vi "Print VI panel to PDF.vi"(6 "jobIndex (0)":i32, 7 "Entire Panel? (T)":bool=TRUE, 8 "error in":errorcluster, 9 "Time out (3 sec)":i32=3, 10 "VI in":refnum<vi>, 11 "path":path) -> (0 "error out":errorcluster, 2 "IsSuccessful":bool, 3 "path out":path)   [LabVIEW 2020]
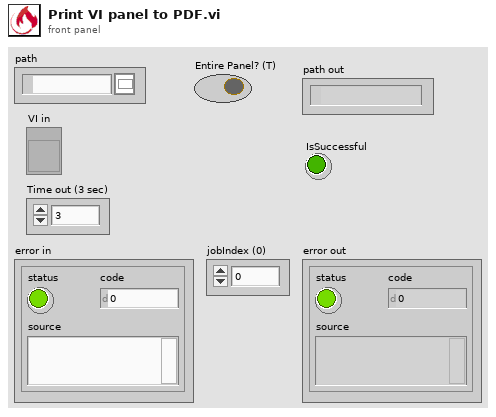
[diagram p1: front panel]
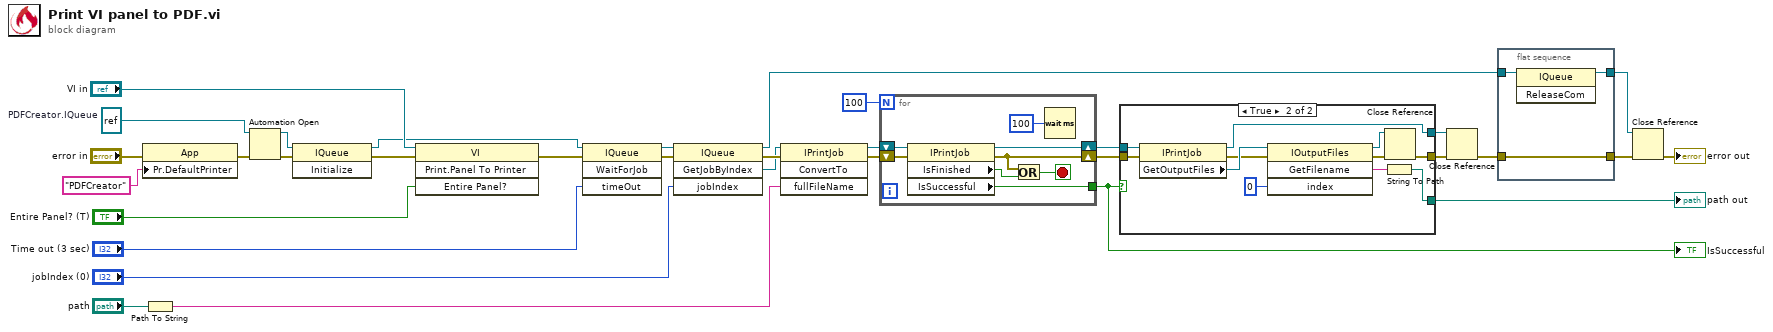
[diagram p0: block diagram]
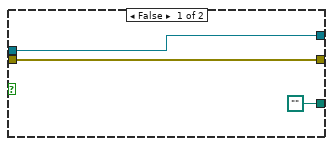
[diagram p2: hidden frame]
diagram:
  w28 = refnum<k7> refnum  # PDFCreator.IQueue
  n1 = property class="App"(error in="error in", "Pr.DefaultPrinter"="PDFCreator" ("Printing:Default Printer")) -> (error out=w29:errorcluster)  [unwired: 1 in, 1 out]
  n2 = Path To String(path="path") -> (string=w32:string)
  n3 = Automation Open(error in (no error)=w29, Automation Refnum=w28) -> (Automation Refnum=w13:refnum<k7>, error out=w14:errorcluster)  [unwired: 2 in]
  n4 = invoke class="IQueue" method="Initialize"(reference=w13, error in=w14) -> (reference out=w15:refnum<k7>, error out=w20:errorcluster)  [unwired: 1 in, 1 out]
  n5 = invoke class="VI" method="Print.Panel To Printer"(reference="VI in", error in=w20, "Entire Panel?"="Entire Panel? (T)") -> (error out=w21:errorcluster)  [unwired: 1 in, 3 out]
  n6 = invoke class="IQueue" method="WaitForJob"(reference=w15, error in=w21, "timeOut"="Time out (3 sec)") -> (reference out=w17:refnum<k7>, error out=w22:errorcluster)  [unwired: 1 in, 2 out]
  n7 = invoke class="IQueue" method="GetJobByIndex"(reference=w17, error in=w22, "jobIndex"="jobIndex (0)") -> (reference out=w11:refnum<k7>, error out=w23:errorcluster, "GetJobByIndex"=w19:refnum<k7>)  [unwired: 1 in, 1 out]
  n8 = invoke class="IPrintJob" method="ConvertTo"(reference=w19, error in=w23, "fullFileName"=w32) -> (reference out=w9:refnum<k7>, error out=w7:errorcluster)  [unwired: 1 in, 2 out]
  n9 = for {
    N: 100 -> [_]
    shift-right: [w40] -> w8
    shift-left: w9 -> [w41]
    shift-right: [w36] -> w5
    shift-left: w7 -> [w39]
    tunnel: [w38] -> w3
    stop <- w34 stop-if-true
    n10 = property class="IPrintJob"(reference=w41, error in=w39) -> (reference out=w40:refnum<k7>, error out=w36:errorcluster, "IsFinished"=w35:bool, "IsSuccessful"=w38:bool)
    n11 = Or(x=w36, y=w35) -> (x .or. y?=w34:bool)
    n12 = Wait (ms)(milliseconds to wait=u32 100) -> ()  [unwired: 1 out]
  }
  "IsSuccessful" <- w3
  n13 = case shown="True" w3 {
    tunnel: [w44 w54] -> w10
    tunnel: w8 -> [w44 w53]
    tunnel: w5 -> [w43 w51]
    tunnel: [w43 w47] -> w4
    tunnel: [path "" w45] -> w1
    frame False {
    }
    frame True {
      n14 = property class="IPrintJob"(reference=w53, error in=w51) -> (reference out=w54:refnum<k7>, error out=w50:errorcluster, "GetOutputFiles"=w55:refnum<k7>)
      n15 = invoke class="IOutputFiles" method="GetFilename"(reference=w55, error in=w50, "index"=0) -> (reference out=w48:refnum<k7>, error out=w49:errorcluster, "GetFilename"=w46:string)  [unwired: 1 in, 1 out]
      n16 = String To Path(string=w46) -> (path=w45:path)
      n17 = Close Reference(reference=w48, error in (no error)=w49) -> (error out=w47:errorcluster)
    }
  }
  "path out" <- w1
  n18 = Close Reference(reference=w10, error in (no error)=w4) -> (error out=w25:errorcluster)
  n19 = flat-sequence {
    tunnel: w11 -> [w58]
    tunnel: [w57] -> w24
    tunnel: [w56] -> w26
    tunnel: w25 -> [w56]
    frame #0 {
      n20 = invoke class="IQueue" method="ReleaseCom"(reference=w58) -> (reference out=w57:refnum<k7>)  [unwired: 2 in, 2 out]
    }
  }
  n21 = Close Reference(reference=w24, error in (no error)=w26) -> (error out=→"error out":errorcluster)
